vi "Write Value (Variant).vi"(7 "field name":string, 8 "error in (no error)":errorcluster, 10 "value":variant, 11 "Value in":refnum<class "Value.lvclass">) -> (0 "error out":errorcluster, 2 "value out":variant, 3 "Value out":refnum<class "Value.lvclass">)   [LabVIEW 2020, in "Value.lvlib" / "Value.lvclass"]
uses:
  Value.lvclass
  cceb9e4b-eb75-48e8-aa55-ce9bdc72e988.vi
  a45a0ea4-a1a3-4c44-a2d0-bd9ac2191226.vi
  c2285a35-9ffd-4e7b-9c27-aea24fb1581d.vi
  8f9649cc-7f21-4ef7-860a-133741f03507.vi
  9a7adfbc-dfd7-46c4-b075-4f0440b83174.vi
  f3df2b06-57d5-4a32-8a6e-a93eab4b8334.vi
  1bea9b6c-c326-4b2e-8e3d-45bf733a9c38.vi
  e383973c-90af-4a51-a4c7-5bbe8c763ef6.vi
  d9fbc47b-4e38-408d-93dd-f03e8c927dfc.vi
  f8e0b90b-c4e6-43ce-b49d-bcdb382c13bb.vi
  878da8d4-af84-4ac8-b8bd-4e3d6f536ca0.vi
  1aa6b969-7b68-4eb2-b836-e13a600a071e.vi
  22b99ade-ebf6-47b9-88b0-a2a84584e77c.vi
  0ecc3a10-4d88-4a3f-8e2b-6d81b1eb2788.vi
  7938dc55-06bb-4f46-98b4-31ec94e48f5a.vi
  9cf4c5a1-706a-4248-a3ee-b4c9f4ce04b3.vi
  17bcbbb4-445b-4ae2-9ca0-bb438421ceb4.vi
  ae889fb9-670a-49f8-b5e5-a0c16fe27676.vi
  76e53dd5-f0c3-4a89-968d-82371d9cf6ec.vi
  bc742d90-07da-41a2-bb0a-7e7b2f4baedd.vi
  9c6bba7f-697c-4d5e-a550-b75ffba85a50.vi
  d17b89b1-25de-4b77-9841-199634659aba.vi
  02c85caf-8b62-432b-a175-5fdc5c038fcc.vi
  db2778e5-0a0b-476e-a616-76c34d6078df.vi
  5a5bdb7c-77ef-45fb-97e8-dbe02cadd076.vi
  03112d84-5c9b-4772-aceb-1428f387a576.vi
  b370053f-91cb-4be5-8525-cb241afcd6fe.vi
  21acc165-9bb3-46db-a53e-93d4eb7e31ab.vi
  a549df2c-920d-4323-ba7c-d4da420400e8.vi
  6d74252b-ad3a-45a7-9484-b3c05cdeac0b.vi
  79192ce2-8dd6-4a70-8822-a4eb65a6aaee.vi
  8a659153-4bf4-400b-b716-4e15b1f2a15f.vi
  1431eaa6-23a1-45b9-a4a3-2693041a1402.vi
  8366b1b6-5195-4a32-8846-ef1dc1edc039.vi
  05adf883-15cd-45cb-9d7e-7746134da8fa.vi
  522d9441-c019-479c-9fbf-718d84229053.vi
  2414d7e0-05f5-4190-ab07-d4c7ba67c6a6.vi
  16fc2f7d-2f3d-48d7-828e-6f1655900f08.vi
  efa8a1d7-3bed-4705-901c-3918d28cffa5.vi
  be3d0229-b834-4748-a57b-b2038c1c1ccb.vi
  26f11cd7-ec94-4004-9a33-110acaed2e3e.vi
  270ebb12-d336-49d8-bcbc-e0196ad89af1.vi
  cc62e3b5-8986-4e79-a38c-535dac47f5c9.vi
  6a645410-e7ef-4ed8-b58d-cdb6402696f2.vi
  21c48d27-f92c-4ff3-9f7e-da22303d9520.vi
  71c37fb2-0984-443b-b7b1-928344430237.vi
  0dfc8336-85bc-4349-aa6f-77eea7d3ae68.vi
  d4fece01-f7e1-4bf9-a8a9-9bacda043edb.vi
  <vilib>/Utility/error.llb/Clear Errors.vi
  <vilib>/Utility/Data Type/Get Type Information.vi
  <vilib>/Utility/Data Type/Get Array Information.vi
  <vilib>/Utility/error.llb/Error Cluster From Error Code.vi
  Get Library Path.vi
  <vilib>/ErrorRing/Error Ring.xnode
  Value.lvlib
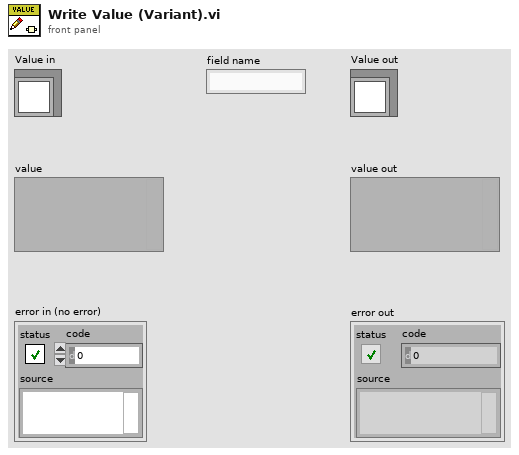
[diagram p1: front panel]
types:
  T1 = typedef "Value.lvlib/Type Code.ctl" = enum8{"Null", "Bool", "BoolA", "Int8", "Int8A", "Int16", "Int16A", "Int32", "Int32A", "Int64", "Int64A", "UInt8", "UInt8A", "UInt16", "UInt16A", "UInt32", "UInt32A", "UInt64", "UInt64A", "Float32", "Float32A", "Float64", "Float64A", "String", "StringA", "Struct", "StructA", "Union", "UnionA", "Any", "AnyA"}
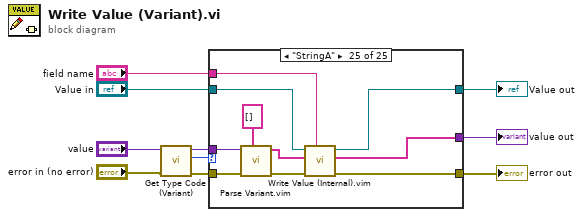
[diagram p0: block diagram]
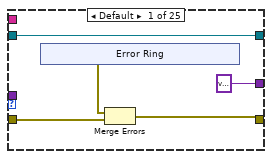
[diagram p2: hidden frame]
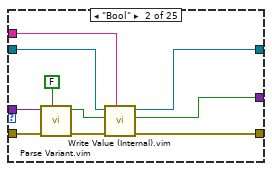
[diagram p3: hidden frame]
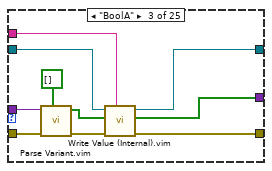
[diagram p4: hidden frame]
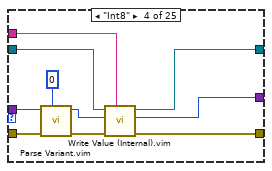
[diagram p5: hidden frame]
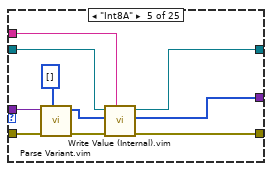
[diagram p6: hidden frame]
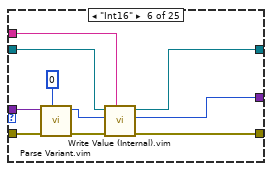
[diagram p7: hidden frame]
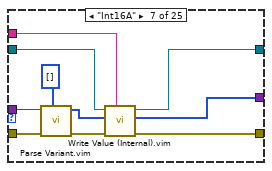
[diagram p8: hidden frame]
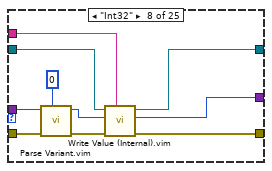
[diagram p9: hidden frame]
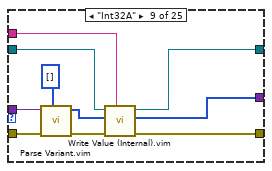
[diagram p10: hidden frame]
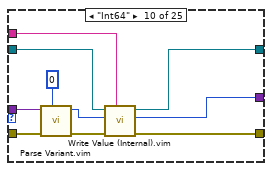
[diagram p11: hidden frame]
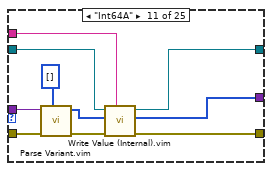
[diagram p12: hidden frame]
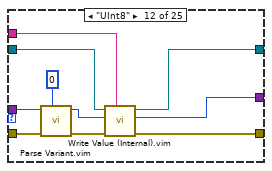
[diagram p13: hidden frame]
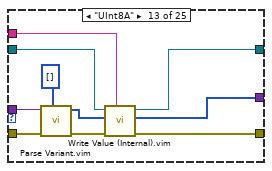
[diagram p14: hidden frame]
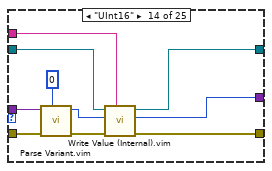
[diagram p15: hidden frame]
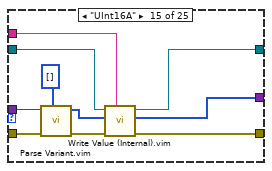
[diagram p16: hidden frame]
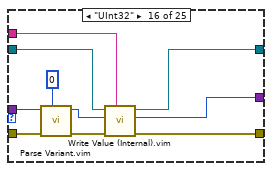
[diagram p17: hidden frame]
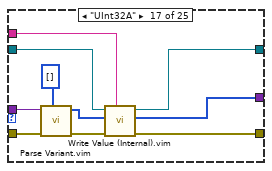
[diagram p18: hidden frame]
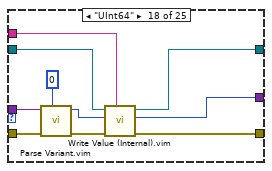
[diagram p19: hidden frame]
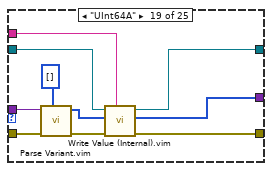
[diagram p20: hidden frame]
diagram:
  n1 = call "Get Type Code (Variant).vi"("error in (no error)"="error in (no error)", "value"="value") -> ("error out"=w8:errorcluster, "type code"=w10:T1, "value dup"=w9:variant)  [unwired: 5 in]
  n2 = case shown="\"StringA\"" w10 {
    tunnel: [w14 w26 w37 w47 w57 w67 w77 w87 w97 w107 w118 w127 w137 w147 w157 w167 w177 w187 w197 w207 w217 w227 w237 w247 w257] -> w4
    tunnel: w8 -> [w15 w29 w39 w49 w59 w69 w79 w89 w99 w109 w119 w129 w139 w149 w159 w169 w179 w189 w199 w209 w219 w229 w239 w249 w259]
    tunnel: [w11 w24 w35 w46 w55 w65 w75 w85 w95 w105 w116 w125 w135 w146 w155 w165 w176 w185 w195 w205 w215 w225 w235 w245 w255] -> w2
    tunnel: w9 -> [_ w23 w34 w45 w54 w64 w74 w84 w94 w104 w115 w124 w134 w145 w154 w164 w175 w184 w194 w204 w214 w224 w234 w244 w254]
    tunnel: [variant w22 w32 w43 w52 w62 w72 w82 w92 w102 w113 w122 w132 w143 w152 w162 w173 w182 w192 w202 w212 w222 w232 w242 w252] -> w5
    tunnel: "Value in" -> [w11 w21 w31 w42 w51 w61 w71 w81 w91 w101 w111 w121 w131 w142 w151 w161 w172 w181 w191 w201 w211 w221 w231 w240 w251]
    tunnel: "field name" -> [_ w20 w30 w40 w50 w60 w70 w80 w90 w100 w110 w120 w130 w140 w150 w160 w170 w180 w190 w200 w210 w220 w230 w241 w250]
    frame Default {
      n3 = xnode "Error Ring"() -> ("error out"=w13:errorcluster)
      n4 = Merge Errors(w13, w15) -> (w14:errorcluster)
    }
    frame "Bool" {
      n5 = call "Parse Variant.vim"("default"=FALSE, "error in (no error)"=w29, "value"=w23) -> ("error out"=w27:errorcluster, "value out"=w25:bool)  [unwired: 7 in]
      n6 = call "Write Value (Internal).vim"("field name"=w20, "error in"=w27, "value"=w25, "Value in"=w21) -> ("error out"=w26:errorcluster, "value out"=w22:bool, "Value out"=w24:refnum<class "Value.lvclass">)  [unwired: 5 in]
    }
    frame "BoolA" {
      n7 = call "Parse Variant.vim"("default"=bool[] [], "error in (no error)"=w39, "value"=w34) -> ("error out"=w38:errorcluster, "value out"=w36:bool[])  [unwired: 7 in]
      n8 = call "Write Value (Internal).vim"("field name"=w30, "error in"=w38, "value"=w36, "Value in"=w31) -> ("error out"=w37:errorcluster, "value out"=w32:bool[], "Value out"=w35:refnum<class "Value.lvclass">)  [unwired: 5 in]
    }
    frame "Int8" {
      n9 = call "Parse Variant.vim"("default"=i8 0, "error in (no error)"=w49, "value"=w45) -> ("error out"=w48:errorcluster, "value out"=w41:i8)  [unwired: 7 in]
      n10 = call "Write Value (Internal).vim"("field name"=w40, "error in"=w48, "value"=w41, "Value in"=w42) -> ("error out"=w47:errorcluster, "value out"=w43:i8, "Value out"=w46:refnum<class "Value.lvclass">)  [unwired: 5 in]
    }
    frame "Int8A" {
      n11 = call "Parse Variant.vim"("default"=i8[] [], "error in (no error)"=w59, "value"=w54) -> ("error out"=w58:errorcluster, "value out"=w56:i8[])  [unwired: 7 in]
      n12 = call "Write Value (Internal).vim"("field name"=w50, "error in"=w58, "value"=w56, "Value in"=w51) -> ("error out"=w57:errorcluster, "value out"=w52:i8[], "Value out"=w55:refnum<class "Value.lvclass">)  [unwired: 5 in]
    }
    frame "Int16" {
      n13 = call "Parse Variant.vim"("default"=i16 0, "error in (no error)"=w69, "value"=w64) -> ("error out"=w68:errorcluster, "value out"=w66:i16)  [unwired: 7 in]
      n14 = call "Write Value (Internal).vim"("field name"=w60, "error in"=w68, "value"=w66, "Value in"=w61) -> ("error out"=w67:errorcluster, "value out"=w62:i16, "Value out"=w65:refnum<class "Value.lvclass">)  [unwired: 5 in]
    }
    frame "Int16A" {
      n15 = call "Parse Variant.vim"("default"=i16[] [], "error in (no error)"=w79, "value"=w74) -> ("error out"=w78:errorcluster, "value out"=w76:i16[])  [unwired: 7 in]
      n16 = call "Write Value (Internal).vim"("field name"=w70, "error in"=w78, "value"=w76, "Value in"=w71) -> ("error out"=w77:errorcluster, "value out"=w72:i16[], "Value out"=w75:refnum<class "Value.lvclass">)  [unwired: 5 in]
    }
    frame "Int32" {
      n17 = call "Parse Variant.vim"("default"=0, "error in (no error)"=w89, "value"=w84) -> ("error out"=w88:errorcluster, "value out"=w86:i32)  [unwired: 7 in]
      n18 = call "Write Value (Internal).vim"("field name"=w80, "error in"=w88, "value"=w86, "Value in"=w81) -> ("error out"=w87:errorcluster, "value out"=w82:i32, "Value out"=w85:refnum<class "Value.lvclass">)  [unwired: 5 in]
    }
    frame "Int32A" {
      n19 = call "Parse Variant.vim"("default"=i32[] [], "error in (no error)"=w99, "value"=w94) -> ("error out"=w98:errorcluster, "value out"=w96:i32[])  [unwired: 7 in]
      n20 = call "Write Value (Internal).vim"("field name"=w90, "error in"=w98, "value"=w96, "Value in"=w91) -> ("error out"=w97:errorcluster, "value out"=w92:i32[], "Value out"=w95:refnum<class "Value.lvclass">)  [unwired: 5 in]
    }
    frame "Int64" {
      n21 = call "Parse Variant.vim"("default"=i64 0, "error in (no error)"=w109, "value"=w104) -> ("error out"=w108:errorcluster, "value out"=w106:i64)  [unwired: 7 in]
      n22 = call "Write Value (Internal).vim"("field name"=w100, "error in"=w108, "value"=w106, "Value in"=w101) -> ("error out"=w107:errorcluster, "value out"=w102:i64, "Value out"=w105:refnum<class "Value.lvclass">)  [unwired: 5 in]
    }
    frame "Int64A" {
      n23 = call "Parse Variant.vim"("default"=i64[] [], "error in (no error)"=w119, "value"=w115) -> ("error out"=w112:errorcluster, "value out"=w117:i64[])  [unwired: 7 in]
      n24 = call "Write Value (Internal).vim"("field name"=w110, "error in"=w112, "value"=w117, "Value in"=w111) -> ("error out"=w118:errorcluster, "value out"=w113:i64[], "Value out"=w116:refnum<class "Value.lvclass">)  [unwired: 5 in]
    }
    frame "UInt8" {
      n25 = call "Parse Variant.vim"("default"=u8 0, "error in (no error)"=w129, "value"=w124) -> ("error out"=w128:errorcluster, "value out"=w126:u8)  [unwired: 7 in]
      n26 = call "Write Value (Internal).vim"("field name"=w120, "error in"=w128, "value"=w126, "Value in"=w121) -> ("error out"=w127:errorcluster, "value out"=w122:u8, "Value out"=w125:refnum<class "Value.lvclass">)  [unwired: 5 in]
    }
    frame "UInt8A" {
      n27 = call "Parse Variant.vim"("default"=u8[] [], "error in (no error)"=w139, "value"=w134) -> ("error out"=w138:errorcluster, "value out"=w136:u8[])  [unwired: 7 in]
      n28 = call "Write Value (Internal).vim"("field name"=w130, "error in"=w138, "value"=w136, "Value in"=w131) -> ("error out"=w137:errorcluster, "value out"=w132:u8[], "Value out"=w135:refnum<class "Value.lvclass">)  [unwired: 5 in]
    }
    frame "UInt16" {
      n29 = call "Parse Variant.vim"("default"=u16 0, "error in (no error)"=w149, "value"=w145) -> ("error out"=w148:errorcluster, "value out"=w141:u16)  [unwired: 7 in]
      n30 = call "Write Value (Internal).vim"("field name"=w140, "error in"=w148, "value"=w141, "Value in"=w142) -> ("error out"=w147:errorcluster, "value out"=w143:u16, "Value out"=w146:refnum<class "Value.lvclass">)  [unwired: 5 in]
    }
    frame "UInt16A" {
      n31 = call "Parse Variant.vim"("default"=u16[] [], "error in (no error)"=w159, "value"=w154) -> ("error out"=w158:errorcluster, "value out"=w156:u16[])  [unwired: 7 in]
      n32 = call "Write Value (Internal).vim"("field name"=w150, "error in"=w158, "value"=w156, "Value in"=w151) -> ("error out"=w157:errorcluster, "value out"=w152:u16[], "Value out"=w155:refnum<class "Value.lvclass">)  [unwired: 5 in]
    }
    frame "UInt32" {
      n33 = call "Parse Variant.vim"("default"=u32 0, "error in (no error)"=w169, "value"=w164) -> ("error out"=w168:errorcluster, "value out"=w166:u32)  [unwired: 7 in]
      n34 = call "Write Value (Internal).vim"("field name"=w160, "error in"=w168, "value"=w166, "Value in"=w161) -> ("error out"=w167:errorcluster, "value out"=w162:u32, "Value out"=w165:refnum<class "Value.lvclass">)  [unwired: 5 in]
    }
    frame "UInt32A" {
      n35 = call "Parse Variant.vim"("default"=u32[] [], "error in (no error)"=w179, "value"=w175) -> ("error out"=w178:errorcluster, "value out"=w171:u32[])  [unwired: 7 in]
      n36 = call "Write Value (Internal).vim"("field name"=w170, "error in"=w178, "value"=w171, "Value in"=w172) -> ("error out"=w177:errorcluster, "value out"=w173:u32[], "Value out"=w176:refnum<class "Value.lvclass">)  [unwired: 5 in]
    }
    frame "UInt64" {
      n37 = call "Parse Variant.vim"("default"=u64 0, "error in (no error)"=w189, "value"=w184) -> ("error out"=w188:errorcluster, "value out"=w186:u64)  [unwired: 7 in]
      n38 = call "Write Value (Internal).vim"("field name"=w180, "error in"=w188, "value"=w186, "Value in"=w181) -> ("error out"=w187:errorcluster, "value out"=w182:u64, "Value out"=w185:refnum<class "Value.lvclass">)  [unwired: 5 in]
    }
    frame "UInt64A" {
      n39 = call "Parse Variant.vim"("default"=u64[] [], "error in (no error)"=w199, "value"=w194) -> ("error out"=w198:errorcluster, "value out"=w196:u64[])  [unwired: 7 in]
      n40 = call "Write Value (Internal).vim"("field name"=w190, "error in"=w198, "value"=w196, "Value in"=w191) -> ("error out"=w197:errorcluster, "value out"=w192:u64[], "Value out"=w195:refnum<class "Value.lvclass">)  [unwired: 5 in]
    }
    frame "Float32" {
      n41 = call "Parse Variant.vim"("default"=sgl 0.0, "error in (no error)"=w209, "value"=w204) -> ("error out"=w208:errorcluster, "value out"=w206:sgl)  [unwired: 7 in]
      n42 = call "Write Value (Internal).vim"("field name"=w200, "error in"=w208, "value"=w206, "Value in"=w201) -> ("error out"=w207:errorcluster, "value out"=w202:sgl, "Value out"=w205:refnum<class "Value.lvclass">)  [unwired: 5 in]
    }
    frame "Float64" {
      n43 = call "Parse Variant.vim"("default"=0.0, "error in (no error)"=w219, "value"=w214) -> ("error out"=w218:errorcluster, "value out"=w216:dbl)  [unwired: 7 in]
      n44 = call "Write Value (Internal).vim"("field name"=w210, "error in"=w218, "value"=w216, "Value in"=w211) -> ("error out"=w217:errorcluster, "value out"=w212:dbl, "Value out"=w215:refnum<class "Value.lvclass">)  [unwired: 5 in]
    }
    frame "Float32A" {
      n45 = call "Parse Variant.vim"("default"=sgl[] [], "error in (no error)"=w229, "value"=w224) -> ("error out"=w228:errorcluster, "value out"=w226:sgl[])  [unwired: 7 in]
      n46 = call "Write Value (Internal).vim"("field name"=w220, "error in"=w228, "value"=w226, "Value in"=w221) -> ("error out"=w227:errorcluster, "value out"=w222:sgl[], "Value out"=w225:refnum<class "Value.lvclass">)  [unwired: 5 in]
    }
    frame "Float64A" {
      n47 = call "Parse Variant.vim"("default"=dbl[] [], "error in (no error)"=w239, "value"=w234) -> ("error out"=w238:errorcluster, "value out"=w236:dbl[])  [unwired: 7 in]
      n48 = call "Write Value (Internal).vim"("field name"=w230, "error in"=w238, "value"=w236, "Value in"=w231) -> ("error out"=w237:errorcluster, "value out"=w232:dbl[], "Value out"=w235:refnum<class "Value.lvclass">)  [unwired: 5 in]
    }
    frame "String" {
      n49 = call "Parse Variant.vim"("default"="", "error in (no error)"=w249, "value"=w244) -> ("error out"=w248:errorcluster, "value out"=w246:string)  [unwired: 7 in]
      n50 = call "Write Value (Internal).vim"("field name"=w241, "error in"=w248, "value"=w246, "Value in"=w240) -> ("error out"=w247:errorcluster, "value out"=w242:string, "Value out"=w245:refnum<class "Value.lvclass">)  [unwired: 5 in]
    }
    frame "StringA" {
      n51 = call "Parse Variant.vim"("default"=string[] [], "error in (no error)"=w259, "value"=w254) -> ("error out"=w258:errorcluster, "value out"=w256:string[])  [unwired: 7 in]
      n52 = call "Write Value (Internal).vim"("field name"=w250, "error in"=w258, "value"=w256, "Value in"=w251) -> ("error out"=w257:errorcluster, "value out"=w252:string[], "Value out"=w255:refnum<class "Value.lvclass">)  [unwired: 5 in]
    }
  }
  "value out" <- w5
  "error out" <- w4
  "Value out" <- w2
